vi "AD7609 Get Nsamples.vi"() -> (1 "Channel volts":dbl[][](array[numeric]), 2 "error out":errorcluster)   [LabVIEW 2015]
uses:
  <vilib>/Instr/_visa.llb/VISA Open Access Mode.ctl
  AD7609 global.vi
panel:
  out "Channel data":cluster{sgl, sgl, sgl[][]}(graph)={0.0, 2.6666667e-05, []}
  # "PN 25/11/2014,  17/08/2015 (check for stop ack)"
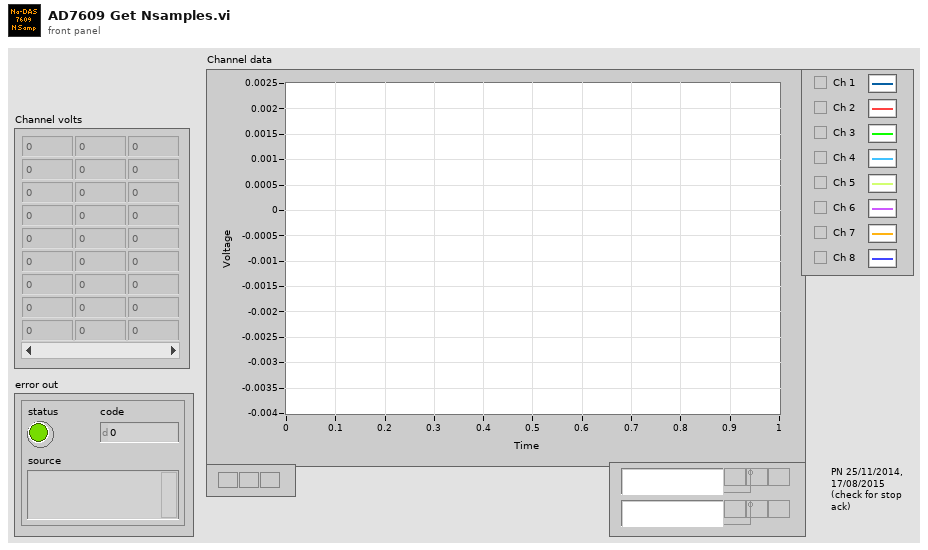
[diagram p1: front panel]
types:
  T1 = typedef "VISA Open Access Mode.ctl" = u32
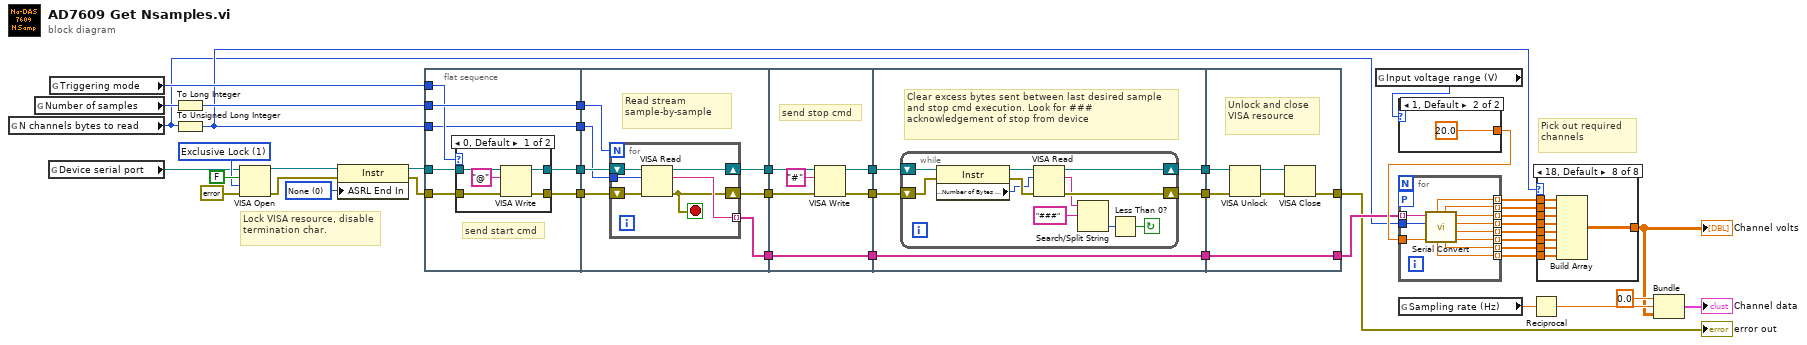
[diagram p0: block diagram]
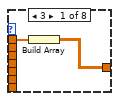
[diagram p2: hidden frame]
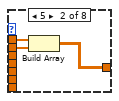
[diagram p3: hidden frame]
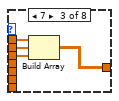
[diagram p4: hidden frame]
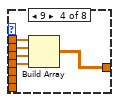
[diagram p5: hidden frame]
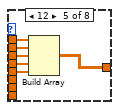
[diagram p6: hidden frame]
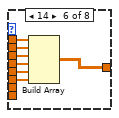
[diagram p7: hidden frame]
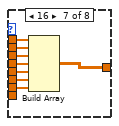
[diagram p8: hidden frame]
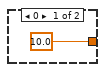
[diagram p9: hidden frame]
diagram:
  w1 = u16 0 items=["None", "Last Bit", "TermChar"] ("Serial Settings:End Mode for Reads")
  w42 = T1 1 items=["VISA Defaults"=0, "Exclusive Lock"=1, "Load Configured Settings"=4] ("Access Mode")
  # "Pick out required channels"
  # "Lock VISA resource, disable termination char."
  n1 = global read "AD7609 global.vi" "N channels bytes to read"() -> (w7:u8)
  n2 = global read "AD7609 global.vi" "Number of samples"() -> (w20:u32)
  n3 = global read "AD7609 global.vi" "Device serial port"() -> (w6:refnum<visa-resource-name>)
  n4 = global read "AD7609 global.vi" "Triggering mode"() -> (w17:u8)
  n5 = To Long Integer(number=w20) -> (32bit integer=w36:i32)
  n6 = To Unsigned Long Integer(number=w7) -> (unsigned 32bit integer=w15:u32)
  n7 = VISA Open(duplicate session (F)=FALSE, access mode=w42, error in (no error)=errorcluster {"status"=FALSE, "code"=0, "source"=""}, VISA resource name=w6) -> (VISA resource name=w5:refnum<visa-resource-name>, error out=w4:errorcluster)  [unwired: 1 in]
  n8 = property class="Instr"(reference=w5, error in=w4, "ASRL End In"=w1) -> (reference out=w3:refnum<visa-resource-name>, error out=w2:errorcluster)
  n9 = flat-sequence {
    tunnel: w2 -> [w51]
    tunnel: w3 -> [w50]
    tunnel: [w49] -> w41
    tunnel: [w48] -> w38
    tunnel: [w47] -> w37
    tunnel: w36 -> [w47]
    tunnel: w17 -> [w46]
    tunnel: w15 -> [w45]
    tunnel: [w45] -> w16
    tunnel: w41 -> [w65]
    tunnel: [w64] -> w40
    tunnel: [w63] -> w39
    tunnel: w38 -> [w62]
    tunnel: w37 -> [w61]
    tunnel: [w60] -> w35
    tunnel: w16 -> [w59]
    tunnel: w40 -> [w76]
    tunnel: w39 -> [w77]
    tunnel: [w73] -> w11
    tunnel: w35 -> [w73]
    tunnel: [w75] -> w12
    tunnel: [w74] -> w13
    tunnel: w13 -> [w78]
    tunnel: w12 -> [w81]
    tunnel: w11 -> [w82]
    tunnel: [w82] -> w10
    tunnel: [w80] -> w9
    tunnel: [w79] -> w8
    tunnel: w10 -> [w96]
    tunnel: [w97] -> w18
    tunnel: [w96] -> w19
    tunnel: w9 -> [w95]
    tunnel: w8 -> [w94]
    frame #0 {
      # "send start cmd"
      n10 = case shown="0, Default" w46 {
        tunnel: w51 -> [w55 w57]
        tunnel: w50 -> [w54 w58]
        tunnel: [w53 w57] -> w49
        tunnel: [w52 w58] -> w48
        frame 0, Default {
          n11 = VISA Write(VISA resource name=w54, write buffer="@", error in (no error)=w55) -> (VISA resource name out=w52:refnum<visa-resource-name>, error out=w53:errorcluster)  [unwired: 1 out]
        }
        frame 1 {
        }
      }
    }
    frame #1 {
      # "Read stream sample-by-sample"
      n12 = for {
        N: w61 -> [_]
        shift-right: [w66] -> w64
        shift-left: w65 -> [w71]
        shift-right: [w70] -> w63
        shift-left: w62 -> [w69]
        tunnel: [w68] -> w60 mode=indexing
        tunnel: w59 -> [w67]
        stop <- w66 stop-if-true
        n13 = VISA Read(VISA resource name=w69, byte count=w67, error in (no error)=w71) -> (VISA resource name out=w70:refnum<visa-resource-name>, read buffer=w68:string, error out=w66:errorcluster)  [unwired: 1 out]
      }
    }
    frame #2 {
      # "send stop cmd"
      n14 = VISA Write(VISA resource name=w77, write buffer="#", error in (no error)=w76) -> (VISA resource name out=w75:refnum<visa-resource-name>, error out=w74:errorcluster)  [unwired: 1 out]
    }
    frame #3 {
      # "Clear excess bytes sent between last desired sample  and stop cmd execution. Look for ### acknowledgement of stop from device"
      n15 = while {
        shift-right: [w89] -> w80
        shift-left: w78 -> [w92]
        shift-right: [w88] -> w79
        shift-left: w81 -> [w93]
        stop <- w84 continue-if-true
        n16 = property class="Instr"(reference=w93, error in=w92) -> (reference out=w91:refnum<visa-resource-name>, error out=w90:errorcluster, "Serial Settings:Number of Bytes at Serial Port"=w83:u32)
        n17 = VISA Read(VISA resource name=w91, byte count=w83, error in (no error)=w90) -> (VISA resource name out=w88:refnum<visa-resource-name>, read buffer=w87:string, error out=w89:errorcluster)  [unwired: 1 out]
        n18 = Search/Split String(string=w87, search string/char (-)="###") -> (offset of match=w85:i32)  [unwired: 1 in, 2 out]
        n19 = Less Than 0?(x=w85) -> (x < 0?=w84:bool)
      }
    }
    frame #4 {
      # "Unlock and close VISA resource"
      n20 = VISA Unlock(8:w95, 11:w94) -> (0:w99:errorcluster, 3:w98:refnum<visa-resource-name>)
      n21 = VISA Close(VISA resource name=w98, error in (no error)=w99) -> (error out=w97:errorcluster)
    }
  }
  n22 = global read "AD7609 global.vi" "Input voltage range (V)"() -> (w30:u8)
  n23 = case shown="1, Default" w30 {
    tunnel: [sgl 10.0 sgl 20.0] -> w31
    frame 0 {
    }
    frame 1, Default {
    }
  }
  n24 = for {
    tunnel: w19 -> [w112] mode=indexing
    tunnel: w31 -> [w111]
    tunnel: [w110] -> w29 mode=indexing
    tunnel: [w109] -> w28 mode=indexing
    tunnel: [w108] -> w27 mode=indexing
    tunnel: [w107] -> w26 mode=indexing
    tunnel: [w106] -> w25 mode=indexing
    tunnel: [w105] -> w24 mode=indexing
    tunnel: [w104] -> w23 mode=indexing
    tunnel: [w103] -> w22 mode=indexing
    workers-P: _ -> [_]
    tunnel: w7 -> [w102]
    n25 = call "Serial Convert.vi"("Range (V)"=w111, "N channels bytes to read"=w102, "Raw serial buffer"=w112) -> ("V6 (V)"=w105:sgl, "V5 (V)"=w106:sgl, "V4 (V)"=w107:sgl, "V3 (V)"=w108:sgl, "V7 (V)"=w104:sgl, "V2 (V)"=w109:sgl, "V8 (V)"=w103:sgl, "V1 (V)"=w110:sgl)  [unwired: 1 in]
  }
  n26 = global read "AD7609 global.vi" "Sampling rate (Hz)"() -> (w33:sgl)
  n27 = Reciprocal(x=w33) -> (1/x=w32:sgl)
  n28 = case shown="18, Default" w15 {
    tunnel: w29 -> [w114 w117 w121 w126 w132 w139 w147 w156]
    tunnel: w28 -> [_ w115 w120 w125 w131 w138 w146 w155]
    tunnel: w27 -> [_ _ w119 w124 w130 w137 w145 w154]
    tunnel: w26 -> [_ _ _ w123 w129 w136 w144 w153]
    tunnel: w25 -> [_ _ _ _ w128 w135 w143 w152]
    tunnel: w24 -> [_ _ _ _ _ w134 w142 w151]
    tunnel: w23 -> [_ _ _ _ _ _ w141 w150]
    tunnel: w22 -> [_ _ _ _ _ _ _ w149]
    tunnel: [w113 w116 w118 w122 w127 w133 w140 w148] -> w21
    frame 3 {
      n29 = Build Array(w114) -> (w113:sgl[][])
    }
    frame 5 {
      n30 = Build Array(w117, w115) -> (w116:sgl[][])
    }
    frame 7 {
      n31 = Build Array(w121, w120, w119) -> (w118:sgl[][])
    }
    frame 9 {
      n32 = Build Array(w126, w125, w124, w123) -> (w122:sgl[][])
    }
    frame 12 {
      n33 = Build Array(w132, w131, w130, w129, w128) -> (w127:sgl[][])
    }
    frame 14 {
      n34 = Build Array(w139, w138, w137, w136, w135, w134) -> (w133:sgl[][])
    }
    frame 16 {
      n35 = Build Array(w147, w146, w145, w144, w143, w142, w141) -> (w140:sgl[][])
    }
    frame 18, Default {
      n36 = Build Array(w156, w155, w154, w153, w152, w151, w150, w149) -> (w148:sgl[][])
    }
  }
  "Channel volts" <- w21
  n37 = Bundle(sgl 0.0, w32, w21) -> (→"Channel data":cluster{sgl, sgl, sgl[][]})  [unwired: 1 in]
  "error out" <- w18
